vi "Update.vi"(8 "error in (no error)":errorcluster, 10 "Engine in":refnum<class "Engine.lvclass">, 11 "DemoGame in":refnum<class "DemoGame.lvclass">) -> (0 "error out":errorcluster, 2 "Engine out":refnum<class "Engine.lvclass">, 3 "DemoGame out":refnum<class "DemoGame.lvclass">)   [LabVIEW 2019, in "RT_Game.lvlib" / "DemoGame.lvclass"]
uses:
  DemoGame.lvclass
  Engine/Engine.lvclass
  Game/Game.lvclass
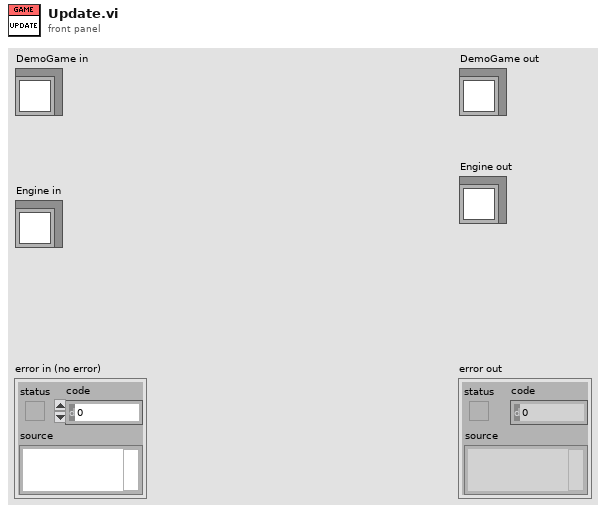
[diagram p1: front panel]
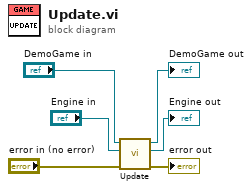
[diagram p0: block diagram]
diagram:
  n1 = call-parent "Update.vi"("error in (no error)"="error in (no error)", "Engine in"="Engine in", "Game in"="DemoGame in") -> ("error out"=→"error out":errorcluster, "Engine out"=→"Engine out":refnum<class "Engine.lvclass">, "Game out"=→"DemoGame out":refnum<class "DemoGame.lvclass">)  [unwired: 6 in]
